vi "CloseOpenRef.vi"(3 "Exp_params":T3={"filename"="201612011532", "ExpFilePath"=path "\\\\10.0.0.7\\takada2/DATA/HBT6/data/Test/201612011532.h5", "File Ref list"=[16777216, 33554432], "sweep_dim"=[4, 2], "sweep_list"=[], "readout_list"=["ADC0", "ADC1"], "Sweep instrument bools"=[[0, 0], [0, 0], [0, 0], [0, 0], [0, 0], [0, 0], [0, 0], [0, 0], [0, 0], [0, 0], [0, 0], [0, 0], [0, 0], [0, 0], [0, 0], [0, 0], [0, 0], [0, 0], [0, 0], [0, 0], [0, 0], [0, 0], [0, 0], [0, 0], [0, 0], [0, 0], [0, 0], [0, 0], [0, 0], [0, 0], [0, 0]], "Read out instrument bools"=[[1, 0]], "Experimental bool list"=[FALSE, TRUE], "Initial move"=[{"Name"="None", "kind"=100, "Value"=0.0}], "FPGA Ref"=refnum, "Inst_parameters"={"ConfigFilePath"=path "\\\\10.0.0.7\\takada2/DATA/HBT6/data/Configs/HBT6_ramp_1.h5", "Inst_list"=["ADC", "AWG", "Freq", "Power", "sus", "rus", "rls", "sls", "suq", "suu", "sur", "suc", "sul", "ruq", "ruu", "rur", "ruc", "rul", "rlq", "rlu", "rlr", "rlc", "rll", "slq", "slu", "slr", "slc", "sll", "tu", "t", "tl", "fast_sequence"], "fast_mode"=[1, 1], "Wait_times"=[1, 1, 1, 1], "Inst_array"=[{"Kind"=0, "Strings"=["ADC", "", "V", "ADC0;ADC1", "V;V", "1.0;1.0"], "uint64s"=[10, 2, 250000, 0, 100, 10106, 1000000, 1, 0, 1], "Doubles"=[1.0], "DAQmx take out list"=[]}, {"Kind"=7, "Strings"=["AWG", "10.0.0.4", "", "C:\\Documents and Settings\\Bauerle\\Mes documents\\Bautze\\FPGA-clean_works_1.13.6_batchtest\\Python\\AWG", "dummy", "SAWnstrig_v4.py"], "uint64s"=[2, 0, 0, 3, 0, 0, 0, 0, 0, 0, 0, 0, 0, 0], "Doubles"=[1200000000.0, 1.0, 0.0, 1.0, 0.0, 1.0, 0.0, 1.0, 0.0, 1.0, 0.0, 1.0, 0.0], "DAQmx take out list"=[]}, {"Kind"=6, "Strings"=["Freq", "0:19", "GHz"], "uint64s"=[1, 0, 0, 0, 2, 0, 0, 0], "Doubles"=[2.0, -30.0, 200.0, 100.0, 0.0, 6.000999927520752, 9.000000318337698e-06, 30.0, -145.0], "DAQmx take out list"=[]}, {"Kind"=6, "Strings"=["Power", "0:19", "GHz"], "uint64s"=[1, 0, 1, 0, 2, 0, 0, 0], "Doubles"=[2.0, -30.0, 200.0, 100.0, 0.0, 6.000999927520752, 9.000000318337698e-06, 30.0, -145.0], "DAQmx take out list"=[]}, {"Kind"=4, "Strings"=["sus", "10.0.0.2", "mV"], "uint64s"=[0, 1], "Doubles"=[1.0, -1.0, 1.0, -1.0, 1.0], "DAQmx take out list"=[]}, {"Kind"=4, "Strings"=["rus", "10.0.0.2", "mV"], "uint64s"=[0, 2], "Doubles"=[1.0, -1.0, 1.0, -1.0, 1.0], "DAQmx take out list"=[]}, {"Kind"=4, "Strings"=["rls", "10.0.0.2", "mV"], "uint64s"=[0, 3], "Doubles"=[1.0, -1.0, 1.0, -1.0, 1.0], "DAQmx take out list"=[]}, {"Kind"=4, "Strings"=["sls", "10.0.0.2", "mV"], "uint64s"=[0, 4], "Doubles"=[1.0, -1.0, 1.0, -1.0, 1.0], "DAQmx take out list"=[]}, {"Kind"=4, "Strings"=["suq", "10.0.0.2", "V"], "uint64s"=[0, 5], "Doubles"=[0.30000001192092896, -2.0, 1.0, -1.0, 1.0], "DAQmx take out list"=[]}, {"Kind"=4, "Strings"=["suu", "10.0.0.2", "V"], "uint64s"=[0, 6], "Doubles"=[0.30000001192092896, -2.0, 1.0, -1.0, 1.0], "DAQmx take out list"=[]}, {"Kind"=4, "Strings"=["sur", "10.0.0.2", "V"], "uint64s"=[0, 7], "Doubles"=[0.30000001192092896, -2.0, 1.0, -1.0, 1.0], "DAQmx take out list"=[]}, {"Kind"=4, "Strings"=["suc", "10.0.0.2", "V"], "uint64s"=[1, 0], "Doubles"=[0.30000001192092896, -2.0, 1.0, -1.0, 1.0], "DAQmx take out list"=[]}, {"Kind"=4, "Strings"=["sul", "10.0.0.2", "V"], "uint64s"=[1, 1], "Doubles"=[0.30000001192092896, -2.0, 1.0, -1.0, 1.0], "DAQmx take out list"=[]}, {"Kind"=4, "Strings"=["ruq", "10.0.0.2", "V"], "uint64s"=[1, 2], "Doubles"=[0.30000001192092896, -2.0, 1.0, -1.0, 1.0], "DAQmx take out list"=[]}, {"Kind"=4, "Strings"=["ruu", "10.0.0.2", "V"], "uint64s"=[1, 3], "Doubles"=[0.30000001192092896, -2.0, 1.0, -1.0, 1.0], "DAQmx take out list"=[]}, {"Kind"=4, "Strings"=["rur", "10.0.0.2", "V"], "uint64s"=[1, 5], "Doubles"=[0.30000001192092896, -2.0, 1.0, -1.0, 1.0], "DAQmx take out list"=[]}, {"Kind"=4, "Strings"=["ruc", "10.0.0.2", "V"], "uint64s"=[1, 6], "Doubles"=[0.30000001192092896, -2.0, 1.0, -1.0, 1.0], "DAQmx take out list"=[]}, {"Kind"=4, "Strings"=["rul", "10.0.0.2", "V"], "uint64s"=[1, 7], "Doubles"=[0.30000001192092896, -2.0, 1.0, -1.0, 1.0], "DAQmx take out list"=[]}, {"Kind"=4, "Strings"=["rlq", "10.0.0.2", "V"], "uint64s"=[2, 0], "Doubles"=[0.30000001192092896, -2.0, 1.0, -1.0, 1.0], "DAQmx take out list"=[]}, {"Kind"=4, "Strings"=["rlu", "10.0.0.2", "V"], "uint64s"=[2, 1], "Doubles"=[0.30000001192092896, -2.0, 1.0, -1.0, 1.0], "DAQmx take out list"=[]}, {"Kind"=4, "Strings"=["rlr", "10.0.0.2", "V"], "uint64s"=[2, 2], "Doubles"=[0.30000001192092896, -2.0, 1.0, -1.0, 1.0], "DAQmx take out list"=[]}, {"Kind"=4, "Strings"=["rlc", "10.0.0.2", "V"], "uint64s"=[2, 3], "Doubles"=[0.30000001192092896, -2.0, 1.0, -1.0, 1.0], "DAQmx take out list"=[]}, {"Kind"=4, "Strings"=["rll", "10.0.0.2", "V"], "uint64s"=[2, 4], "Doubles"=[0.30000001192092896, -2.0, 1.0, -1.0, 1.0], "DAQmx take out list"=[]}, {"Kind"=4, "Strings"=["slq", "10.0.0.2", "V"], "uint64s"=[2, 5], "Doubles"=[0.30000001192092896, -2.0, 1.0, -1.0, 1.0], "DAQmx take out list"=[]}, {"Kind"=4, "Strings"=["slu", "10.0.0.2", "V"], "uint64s"=[2, 6], "Doubles"=[0.30000001192092896, -2.0, 1.0, -1.0, 1.0], "DAQmx take out list"=[]}, {"Kind"=4, "Strings"=["slr", "10.0.0.2", "V"], "uint64s"=[2, 7], "Doubles"=[0.30000001192092896, -2.0, 1.0, -1.0, 1.0], "DAQmx take out list"=[]}, {"Kind"=4, "Strings"=["slc", "10.0.0.2", "V"], "uint64s"=[3, 0], "Doubles"=[0.30000001192092896, -2.0, 1.0, -1.0, 1.0], "DAQmx take out list"=[]}, {"Kind"=4, "Strings"=["sll", "10.0.0.2", "V"], "uint64s"=[3, 1], "Doubles"=[0.30000001192092896, -2.0, 1.0, -1.0, 1.0], "DAQmx take out list"=[]}, {"Kind"=4, "Strings"=["tu", "10.0.0.2", "V"], "uint64s"=[3, 2], "Doubles"=[0.30000001192092896, -2.0, 1.0, -1.0, 1.0], "DAQmx take out list"=[]}, {"Kind"=4, "Strings"=["t", "10.0.0.2", "V"], "uint64s"=[3, 3], "Doubles"=[0.30000001192092896, -2.0, 1.0, -1.0, 1.0], "DAQmx take out list"=[]}, {"Kind"=4, "Strings"=["tl", "10.0.0.2", "V"], "uint64s"=[3, 4], "Doubles"=[0.30000001192092896, -2.0, 1.0, -1.0, 1.0], "DAQmx take out list"=[]}, {"Kind"=9, "Strings"=["fast_sequence", "10.0.0.2", "V"], "uint64s"=[6661, 300, 200, 0, 0, 1, 2, 3, 4, 5, 6, 7, 16, 17, 18, 19, 20, 21, 22, 23, 0], "Doubles"=[0.5, -0.5, -1.0, -1.0], "DAQmx take out list"=[]}]}} {"File Ref list" format="%.0x"}) -> (0 "Exp_params_out":T3 {"File Ref list" format="%.0x"}, 1 "group out":T1 format="%.0x")   [LabVIEW 2010]
uses:
  <vilib>/addons/h5labview2/base/hid_t.ctl
  fpga-bitfile-ref.ctl
  <vilib>/addons/h5labview2/file/H5Fmode.ctl
  <vilib>/addons/h5labview2/group/H5G.lvlib
  <vilib>/addons/h5labview2/file/H5F.lvlib
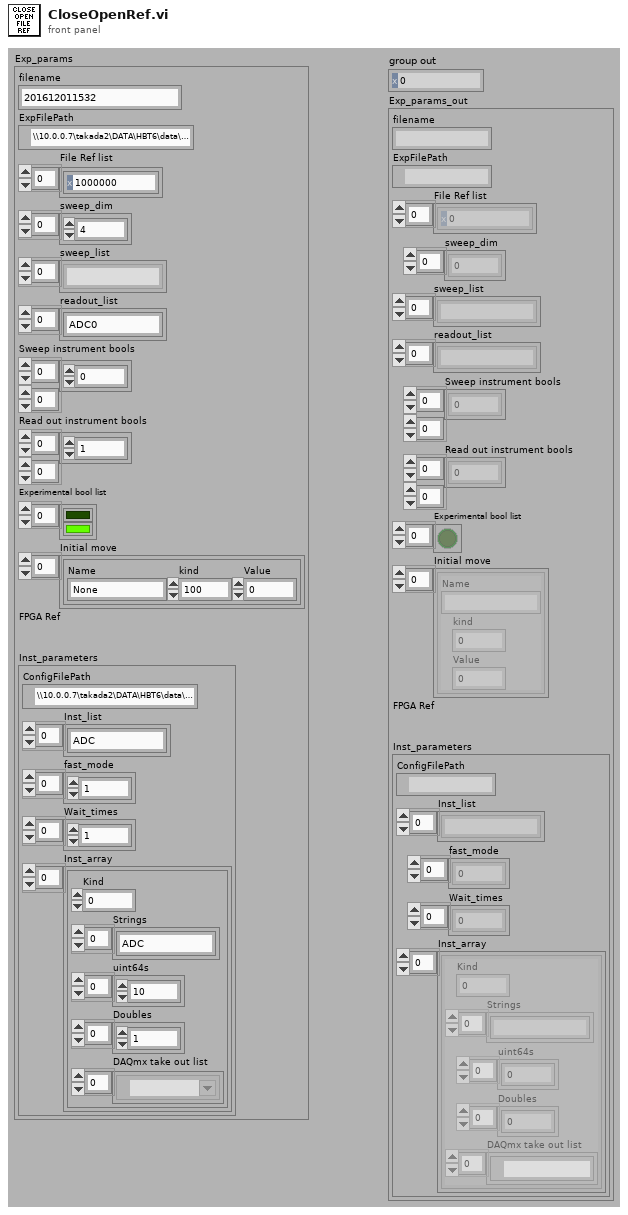
[diagram p1: front panel]
types:
  T1 = typedef "hid_t.ctl" = i32
  T2 = typedef "fpga-bitfile-ref.ctl" = refnum<k20>
  T3 = cluster{"filename":string, "ExpFilePath":path, "File Ref list":T1[], "sweep_dim":u64[], "sweep_list":string[], "readout_list":string[], "Sweep instrument bools":u64[][], "Read out instrument bools":u64[][], "Experimental bool list":bool[], "Initial move":cluster{"Name":string, "kind":u64, "Value":dbl}[], "FPGA Ref":T2, "Inst_parameters":cluster{"ConfigFilePath":path, "Inst_list":string[], "fast_mode":u8[], "Wait_times":u64[], "Inst_array":cluster{"Kind":u16, "Strings":string[], "uint64s":u64[], "Doubles":dbl[], "DAQmx take out list":refnum<k21>[]}[]}}
  T4 = typedef "H5F.lvlib/H5Fmode.ctl" = enum16{"read-only", "read-write", "overwrite", "create new", "open or create"}
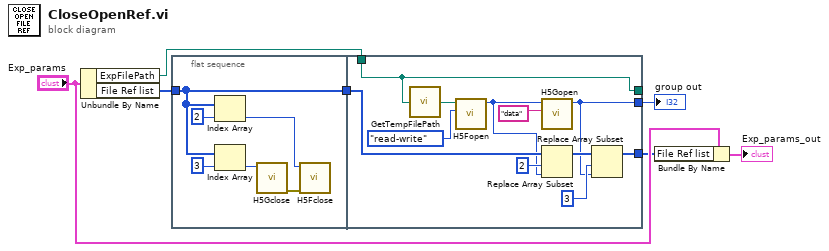
[diagram p0: block diagram]
diagram:
  n1 = Unbundle By Name("Exp_params") -> ("ExpFilePath"=w5:path, "File Ref list"=w6:T1[])
  n2 = flat-sequence {
    tunnel: w6 -> [w8]
    tunnel: [w8] -> w7
    tunnel: w7 -> [w20]
    tunnel: [w24] -> _
    tunnel: w5 -> [w24]
    tunnel: [w15] -> w3
    tunnel: [w14] -> w2
    frame #0 {
      n3 = Index Array(array=w8, index=2) -> (element=w9:T1)
      n4 = Index Array(array=w8, index=3) -> (element=w10:T1)
      n5 = call <vilib>:"H5Gclose.vi"("group in"=w10) -> ("error out"=w13:errorcluster)  [unwired: 10 in]
      n6 = call <vilib>:"H5Fclose.vi"("error in (no error)"=w13, "ref"=w9) -> ()  [unwired: 9 in, 1 out]
    }
    frame #1 {
      n7 = call "GetTempFilePath.vi"("ExpFilePath"=w24) -> ("Temp file path"=w23:path)
      n8 = call <vilib>:"H5Fopen.vi"("mode (read-only)"=H5Fmode."read-write" ("mode"), "path"=w23) -> ("ref out"=w16:T1)  [unwired: 8 in, 1 out]
      n9 = call <vilib>:"H5Gopen.vi"("name"="data", "ref in"=w16) -> ("group out"=w14:T1)  [unwired: 8 in, 1 out]
      n10 = Replace Array Subset(array=w20, new element=w16, index=2) -> (w19:T1[])
      n11 = Replace Array Subset(array=w19, new element=w14, index=3) -> (w15:T1[])
    }
  }
  n12 = Bundle By Name(cluster="Exp_params", "File Ref list"=w3) -> (→"Exp_params_out":T3)
  "group out" <- w2
